vi "update engine info names.vi"(8 "error in":errorcluster, 10 "engine in":refnum<class "Engine Parent Editor Node.lvclass">, 11 "shared memory editor node in":refnum<class "module editor node.lvclass">) -> (0 "error out":errorcluster, 2 "engine out":refnum<class "Engine Parent Editor Node.lvclass">, 3 "shared memory editor node out":refnum<class "module editor node.lvclass">)   [LabVIEW 2014, in "Shared Memory editor node.lvclass"]
uses:
  Shared Memory editor node.lvclass
  <vilib>/NI/DCAF/Tag Editor Core/Configuration Editor/Classes/Module editor node/module editor node.lvclass
  <vilib>/NI/DCAF/Tag Editor Core/Configuration Editor/Classes/Engine Parent/Engine Parent Editor Node.lvclass
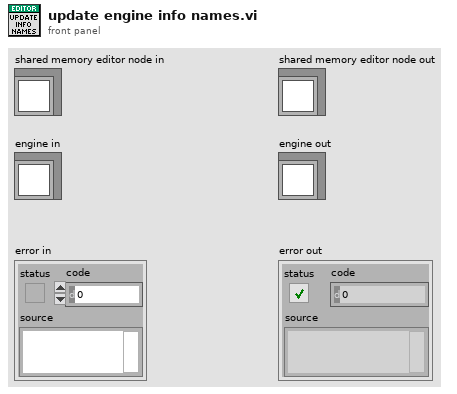
[diagram p1: front panel]
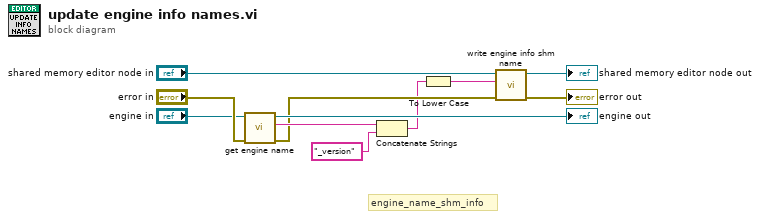
[diagram p0: block diagram]
diagram:
  # "engine_name_shm_info"
  n1 = call "get engine name.vi"("error in (no error)"="error in", "engine in"="engine in") -> ("error out"=w4:errorcluster, "engine name"=w7:string, "engine out"=→"engine out":refnum<class "Engine Parent Editor Node.lvclass">)  [unwired: 7 in]
  n2 = Concatenate Strings(w7, "_version" ("string")) -> (w1:string)
  n3 = To Lower Case(string=w1) -> (all lower case string=w2:string)
  n4 = call "write engine info shm name.vi"("error in"=w4, "shm name"=w2, "shared memory editor node"="shared memory editor node in") -> ("error out"=→"error out":errorcluster, "shared memory editor node out"=→"shared memory editor node out":refnum<class "module editor node.lvclass">)  [unwired: 7 in]
